vi "DSF.Engine.Runtime.Set Timing.vi"(8 "error in (no error)":errorcluster, 10 "Timing":refnum<class "DSF.Shared.Timing.lvclass">, 11 "Runtime in":refnum<class "DSF.Engine.Runtime.lvclass">) -> (0 "error out":errorcluster, 3 "Runtime out":refnum<class "DSF.Engine.Runtime.lvclass">)   [LabVIEW 2017, in "DSF.Engine.lvlib" / "DSF.Engine.Runtime.lvclass"]
uses:
  DSF.Engine.Runtime.lvclass
  Shared/Classes/Timing/DSF.Shared.Timing.lvclass
  DSF.Engine.Runtime.lvclass/DSF.Engine.Runtime.ctl
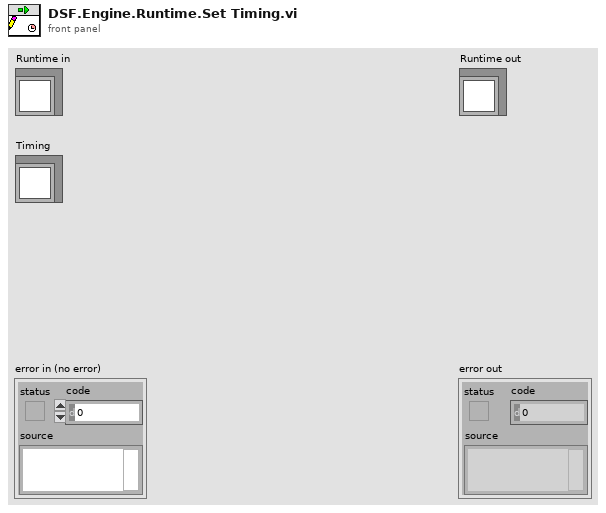
[diagram p1: front panel]
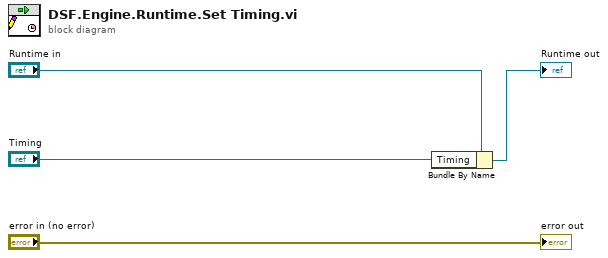
[diagram p0: block diagram]
diagram:
  n1 = Bundle By Name(cluster="Runtime in", "Timing"="Timing") -> (→"Runtime out":refnum<class "DSF.Engine.Runtime.lvclass">)
  "error out" <- "error in (no error)"
